vi "Reset Output(SubVI).vi"(8 "error in (no error)":errorcluster, 9 "WFGraph Refnum 2":refnum<vi>, 10 "WFGraph Refnum":refnum<vi>, 11 "Cluster in":refnum<vi>) -> (0 "error out":errorcluster)   [LabVIEW 2018]
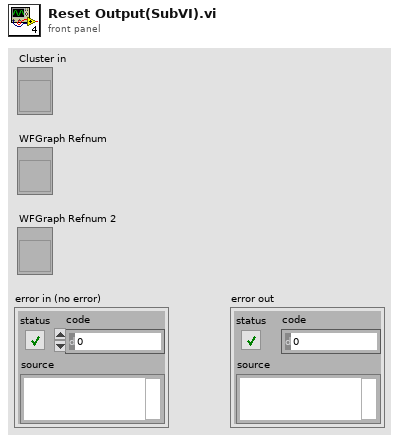
[diagram p1: front panel]
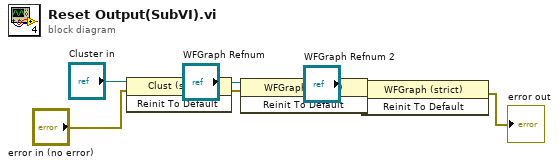
[diagram p0: block diagram]
diagram:
  n1 = invoke on="Invoke Node" class="Clust (strict)" method="Reinit To Default"(reference="Cluster in", error in="error in (no error)") -> (error out=w5:errorcluster)  [unwired: 1 in, 2 out]
  n2 = invoke on="Invoke Node" class="WFGraph (strict)" method="Reinit To Default"(reference="WFGraph Refnum", error in=w5) -> (error out=w6:errorcluster)  [unwired: 1 in, 2 out]
  n3 = invoke on="Invoke Node" class="WFGraph (strict)" method="Reinit To Default"(reference="WFGraph Refnum 2", error in=w6) -> (error out=→"error out":errorcluster)  [unwired: 1 in, 2 out]
